vi "Map Memory.vi"(8 "error in (no error)":errorcluster, 9 "process (shared)":T1, 10 "protections (read/write)":T2={"read"=TRUE, "write"=TRUE, "execute"=FALSE}, 11 "Shared Memory in":refnum<class "Shared Memory.lvclass">) -> (0 "error out":errorcluster, 2 "pointer":u64, 3 "Shared Memory out":refnum<class "Shared Memory.lvclass">)   [LabVIEW 2013, in "Linux RT IPC.Shared Memory.lvlib" / "Shared Memory.lvclass"]
doc: "This VI calls the mmap() function using the currently open file descriptor and stores the returned pointer value in the class member data."
uses:
  Shared Memory.lvclass
  C/Controls/mman sharing.ctl
  Shared Memory.lvclass/Shared Memory.ctl
  C/SubVIs/error handler.vi
  <vilib>/NI/NI Linux RT Errno/VIs/Public/Get Errno Value for Calling Thread.vi
  C/Linux RT IPC.C.lvlib
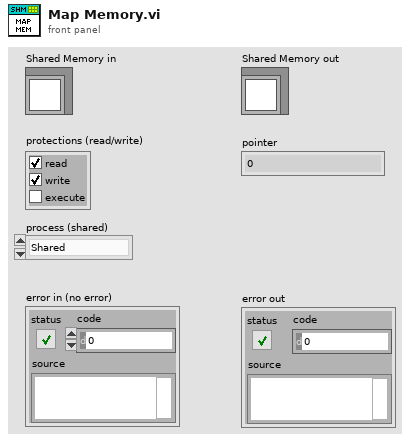
[diagram p1: front panel]
types:
  T1 = typedef "Linux RT IPC.C.lvlib/mman sharing.ctl" = enum16{"Shared", "Private"}
  T2 = cluster{"read":bool, "write":bool, "execute":bool}
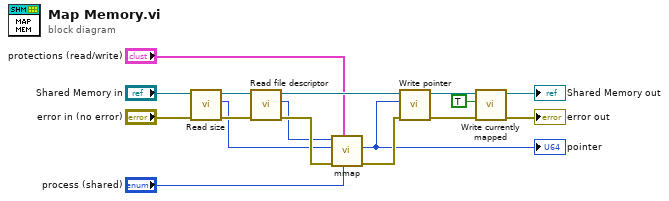
[diagram p0: block diagram]
diagram:
  n1 = call "Read size.vi"("error in (no error)"="error in (no error)", "Shared Memory in"="Shared Memory in") -> ("error out"=w10:errorcluster, "size (bytes)"=w4:u64, "Shared Memory out"=w8:refnum<class "Shared Memory.lvclass">)  [unwired: 7 in]
  n2 = call "Read file descriptor.vi"("error in (no error)"=w10, "Shared Memory in"=w8) -> ("error out"=w6:errorcluster, "file descriptor"=w5:i32, "Shared Memory out"=w11:refnum<class "Shared Memory.lvclass">)  [unwired: 7 in]
  n3 = call "mmap.vi"("process (shared)"="process (shared)", "protections (read/write)"="protections (read/write)", "error in (no error)"=w6, "number of bytes"=w4, "file descriptor"=w5) -> ("error out"=w12:errorcluster, "pointer"=w3:u64)  [unwired: 4 in, 1 out]
  "pointer" <- w3
  n4 = call "Write pointer.vi"("error in (no error)"=w12, "pointer"=w3, "Shared Memory in"=w11) -> ("error out"=w14:errorcluster, "Shared Memory out"=w13:refnum<class "Shared Memory.lvclass">)  [unwired: 7 in]
  n5 = call "Write currently mapped.vi"("error in (no error)"=w14, "currently mapped"=TRUE, "Shared Memory in"=w13) -> ("error out"=→"error out":errorcluster, "Shared Memory out"=→"Shared Memory out":refnum<class "Shared Memory.lvclass">)  [unwired: 7 in]
